vi "BMU诊断标定.vi"(5 "timeout":u32, 6 "Socket":dbl, 7 "通用配置?":bool, 8 "CAN端口":u16(ring), 9 "设备索引号":u16(ring), 10 "CAN卡类型":u32(ring)=21, 11 "从板号":u8=1) -> (3 "成功?":bool)   [LabVIEW 2013] (continued)
                n1293 = property on="配置文件版本" class="Str"("Disabled"=w1973) -> ()  [unwired: 2 in, 2 out]
                n1294 = property on="车架(牌)号" class="Str"("Disabled"=w1973) -> ()  [unwired: 2 in, 2 out]
                n1295 = property on="项目信息2" class="Clust (严格)"("DisabledEnum"=w1973) -> ()  [unwired: 2 in, 2 out]
                n1296 = property on="产品编号" class="Str"("Disabled"=w1973) -> ()  [unwired: 2 in, 2 out]
                n1297 = Not(x=w1977) -> (.not. x?=w1976:bool)
              }
              frame "产品编号" {
                w1990 = 2
                w1992 = FALSE
                n1298 = property on="项目信息" class="Tbl (严格)"("Disabled"=w1990) -> ()  [unwired: 2 in, 2 out]
                n1299 = property on="电池实际容量(A)" class="DigNum (严格)"("Disabled"=w1990) -> ()  [unwired: 2 in, 2 out]
                n1300 = property on="使用者" class="DigNum (严格)"("Disabled"=w1990) -> ()  [unwired: 2 in, 2 out]
                n1301 = Select(t=0, s=w1981, f=1) -> (s? t:f=w1980:i32)
                n1302 = property on="SOH(%)" class="DigNum (严格)"("Disabled"=w1990) -> ()  [unwired: 2 in, 2 out]
                n1303 = property on="电池额定容量(A)" class="DigNum (严格)"("Disabled"=w1990) -> ()  [unwired: 2 in, 2 out]
                n1304 = property on="SOC(%)" class="DigNum (严格)"("Disabled"=w1990) -> ()  [unwired: 2 in, 2 out]
                n1305 = property on="产品编号" class="Str"("Disabled"=w1980) -> ()  [unwired: 2 in, 2 out]
                n1306 = property on="项目信息2" class="Clust (严格)"("DisabledEnum"=w1980) -> ()  [unwired: 2 in, 2 out]
                n1307 = property on="系统时钟" class="Str"("Disabled"=w1990) -> ()  [unwired: 2 in, 2 out]
                n1308 = property on="配置文件版本" class="Str"("Disabled"=w1990) -> ()  [unwired: 2 in, 2 out]
                n1309 = property on="车架(牌)号" class="Str"("Disabled"=w1990) -> ()  [unwired: 2 in, 2 out]
                n1310 = property on="从板个数" class="DigNum (严格)"("NumText.BGColor"=u32 13816530) -> ()  [unwired: 2 in, 2 out]
                n1311 = global read "功能码全局.vi" "主板项目信息5"() -> (w1988:bool[])
                n1312 = global read "功能码全局.vi" "主板项目信息6"() -> (w1985:bool[])
                n1313 = Index Array(array=w1988, index=0 ("索引")) -> (element=w1987:bool)
                n1314 = Index Array(array=w1985, index=1 ("索引")) -> (element=w1984:bool)
                n1315 = Not(x=w1992) -> (.not. x?=w1991:bool)
              }
              frame "电压个数" {
                w2007 = 2
                w2009 = FALSE
                n1316 = local read "从板个数"() -> (w2006:dbl)
                n1317 = property on="从板个数" class="DigNum (严格)"("NumText.BGColor"=u32 6618880) -> ()  [unwired: 2 in, 2 out]
                n1318 = property on="电池实际容量(A)" class="DigNum (严格)"("Disabled"=w2007) -> ()  [unwired: 2 in, 2 out]
                n1319 = property on="使用者" class="DigNum (严格)"("Disabled"=w2007) -> ()  [unwired: 2 in, 2 out]
                n1320 = property on="SOH(%)" class="DigNum (严格)"("Disabled"=w2007) -> ()  [unwired: 2 in, 2 out]
                n1321 = property on="电池额定容量(A)" class="DigNum (严格)"("Disabled"=w2007) -> ()  [unwired: 2 in, 2 out]
                n1322 = property on="SOC(%)" class="DigNum (严格)"("Disabled"=w2007) -> ()  [unwired: 2 in, 2 out]
                n1323 = property on="系统时钟" class="Str"("Disabled"=w2007) -> ()  [unwired: 2 in, 2 out]
                n1324 = property on="配置文件版本" class="Str"("Disabled"=w2007) -> ()  [unwired: 2 in, 2 out]
                n1325 = property on="车架(牌)号" class="Str"("Disabled"=w2007) -> ()  [unwired: 2 in, 2 out]
                n1326 = property on="产品编号" class="Str"("Disabled"=w2007) -> ()  [unwired: 2 in, 2 out]
                n1327 = Select(t=0, s=w1996, f=1) -> (s? t:f=w1995:i32)
                n1328 = control-ref of="项目信息"() -> (w2005:refnum<vi>)
                n1329 = stacked-sequence {
                  tunnel: w2006 -> [_ w2016 w2026]
                  tunnel: w2005 -> [w2011 w2015 w2027]
                  frame #0 {
                    w2012 = 0
                    n1330 = Bundle(w2012, w2012) -> (w2014:cluster{i32, i32})  [unwired: 1 out]
                    n1331 = property class="Tbl (严格)"(reference=w2011, "Index Values"=w2014) -> (error out=w2013:errorcluster)  [unwired: 1 in, 1 out]
                    n1332 = call <vilib>:"Clear Errors.vi"("error in (no error)"=w2013) -> ()  [unwired: 7 out]
                  }
                  frame #1 {
                    n1333 = for {
                      N: 10 -> [_]
                      tunnel: w2015 -> [w2025]
                      tunnel: w2016 -> [w2020]
                      i -> [w2019]
                      n1334 = Compound Arithmetic op=ADD(0.0 ("值"), w2020, w2019) -> (w2022:dbl)
                      n1335 = Bundle(w2022, 0) -> (w2024:cluster{dbl, i32})  [unwired: 1 out]
                      n1336 = property class="Tbl (严格)"(reference=w2025, "Active Cell"=w2024, "Cell BG Color"=u32 16448250) -> ()  [unwired: 1 in, 2 out]
                    }
                  }
                  frame #2 {
                    n1337 = for {
                      N: w2026 -> [_]
                      tunnel: w2027 -> [w2028]
                      i -> [w2029]
                      n1338 = Bundle(w2029, 0) -> (w2033:cluster{i32, i32})  [unwired: 1 out]
                      n1339 = property class="Tbl (严格)"(reference=w2028, "Active Cell"=w2033, "Cell BG Color"=u32 6618880) -> (error out=w2030:errorcluster)  [unwired: 1 in, 1 out]
                      n1340 = call <vilib>:"Clear Errors.vi"("error in (no error)"=w2030) -> ()  [unwired: 7 out]
                    }
                  }
                }
                n1341 = property on="项目信息" class="Tbl (严格)"("Disabled"=w1995) -> ()  [unwired: 2 in, 2 out]
                n1342 = global read "功能码全局.vi" "主板项目信息5"() -> (w2003:bool[])
                n1343 = global read "功能码全局.vi" "主板项目信息6"() -> (w2001:bool[])
                n1344 = Index Array(array=w2003, index=1 ("索引")) -> (element=w2000:bool)
                n1345 = Index Array(array=w2001, index=2 ("索引")) -> (element=w1999:bool)
                n1346 = Not(x=w2009) -> (.not. x?=w2008:bool)
              }
              frame "通道电压数" {
                w2047 = 2
                w2049 = FALSE
                n1347 = property on="从板个数" class="DigNum (严格)"("NumText.BGColor"=u32 13816530) -> ()  [unwired: 2 in, 2 out]
                n1348 = property on="电池实际容量(A)" class="DigNum (严格)"("Disabled"=w2047) -> ()  [unwired: 2 in, 2 out]
                n1349 = property on="使用者" class="DigNum (严格)"("Disabled"=w2047) -> ()  [unwired: 2 in, 2 out]
                n1350 = property on="SOH(%)" class="DigNum (严格)"("Disabled"=w2047) -> ()  [unwired: 2 in, 2 out]
                n1351 = property on="电池额定容量(A)" class="DigNum (严格)"("Disabled"=w2047) -> ()  [unwired: 2 in, 2 out]
                n1352 = property on="SOC(%)" class="DigNum (严格)"("Disabled"=w2047) -> ()  [unwired: 2 in, 2 out]
                n1353 = local read "从板个数"() -> (w2045:dbl)
                n1354 = property on="系统时钟" class="Str"("Disabled"=w2047) -> ()  [unwired: 2 in, 2 out]
                n1355 = property on="配置文件版本" class="Str"("Disabled"=w2047) -> ()  [unwired: 2 in, 2 out]
                n1356 = property on="车架(牌)号" class="Str"("Disabled"=w2047) -> ()  [unwired: 2 in, 2 out]
                n1357 = property on="产品编号" class="Str"("Disabled"=w2047) -> ()  [unwired: 2 in, 2 out]
                n1358 = control-ref of="项目信息"() -> (w2046:refnum<vi>)
                n1359 = stacked-sequence {
                  tunnel: w2046 -> [w2056 w2059]
                  tunnel: w2045 -> [w2055 w2058]
                  frame #0 {
                    n1360 = Compound Arithmetic op=ADD(1.0 ("值"), w2055) -> (w2052:dbl)
                    n1361 = Bundle(w2052, 0) -> (w2054:cluster{dbl, i32})  [unwired: 1 out]
                    n1362 = property class="Tbl (严格)"(reference=w2056, "Index Values"=w2054) -> ()  [unwired: 1 in, 2 out]
                  }
                  frame #1 {
                    n1363 = for {
                      N: 20 -> [_]
                      tunnel: w2059 -> [w2067]
                      tunnel: w2058 -> [w2062]
                      i -> [w2061]
                      n1364 = Compound Arithmetic op=ADD(1.0 ("值"), w2062, w2061) -> (w2064:dbl)
                      n1365 = Bundle(w2064, 0) -> (w2066:cluster{dbl, i32})  [unwired: 1 out]
                      n1366 = property class="Tbl (严格)"(reference=w2067, "Active Cell"=w2066, "Cell BG Color"=u32 6618880) -> ()  [unwired: 1 in, 2 out]
                    }
                  }
                }
                n1367 = Select(t=0, s=w2035, f=1) -> (s? t:f=w2036:i32)
                n1368 = property on="项目信息" class="Tbl (严格)"("Disabled"=w2036) -> ()  [unwired: 2 in, 2 out]
                n1369 = global read "功能码全局.vi" "主板项目信息5"() -> (w2043:bool[])
                n1370 = global read "功能码全局.vi" "主板项目信息6"() -> (w2041:bool[])
                n1371 = Index Array(array=w2043, index=2 ("索引")) -> (element=w2040:bool)
                n1372 = Index Array(array=w2041, index=3 ("索引")) -> (element=w2039:bool)
                n1373 = Not(x=w2049) -> (.not. x?=w2048:bool)
              }
              frame "电压起始值" {
                w2081 = 2
                w2083 = FALSE
                n1374 = property on="从板个数" class="DigNum (严格)"("NumText.BGColor"=u32 13816530) -> ()  [unwired: 2 in, 2 out]
                n1375 = property on="电池实际容量(A)" class="DigNum (严格)"("Disabled"=w2081) -> ()  [unwired: 2 in, 2 out]
                n1376 = property on="使用者" class="DigNum (严格)"("Disabled"=w2081) -> ()  [unwired: 2 in, 2 out]
                n1377 = property on="SOH(%)" class="DigNum (严格)"("Disabled"=w2081) -> ()  [unwired: 2 in, 2 out]
                n1378 = property on="电池额定容量(A)" class="DigNum (严格)"("Disabled"=w2081) -> ()  [unwired: 2 in, 2 out]
                n1379 = property on="SOC(%)" class="DigNum (严格)"("Disabled"=w2081) -> ()  [unwired: 2 in, 2 out]
                n1380 = local read "从板个数"() -> (w2079:dbl)
                n1381 = property on="系统时钟" class="Str"("Disabled"=w2081) -> ()  [unwired: 2 in, 2 out]
                n1382 = property on="配置文件版本" class="Str"("Disabled"=w2081) -> ()  [unwired: 2 in, 2 out]
                n1383 = property on="车架(牌)号" class="Str"("Disabled"=w2081) -> ()  [unwired: 2 in, 2 out]
                n1384 = property on="产品编号" class="Str"("Disabled"=w2081) -> ()  [unwired: 2 in, 2 out]
                n1385 = control-ref of="项目信息"() -> (w2080:refnum<vi>)
                n1386 = stacked-sequence {
                  tunnel: w2080 -> [w2090 w2093 w2106]
                  tunnel: w2079 -> [w2089 w2092 w2105]
                  frame #0 {
                    n1387 = Compound Arithmetic op=ADD(21.0 ("值"), w2089) -> (w2086:dbl)
                    n1388 = Bundle(w2086, 0) -> (w2088:cluster{dbl, i32})  [unwired: 1 out]
                    n1389 = property class="Tbl (严格)"(reference=w2090, "Index Values"=w2088) -> ()  [unwired: 1 in, 2 out]
                  }
                  frame #1 {
                    n1390 = for {
                      N: 10 -> [_]
                      tunnel: w2093 -> [w2103]
                      tunnel: w2092 -> [w2098]
                      i -> [w2097]
                      n1391 = Multiply(x=w2098, y=2.0) -> (x*y=w2095:dbl)
                      n1392 = Compound Arithmetic op=ADD(21.0 ("值"), w2095, w2097) -> (w2100:dbl)
                      n1393 = Bundle(w2100, 0) -> (w2102:cluster{dbl, i32})  [unwired: 1 out]
                      n1394 = property class="Tbl (严格)"(reference=w2103, "Active Cell"=w2102, "Cell BG Color"=u32 16448250) -> ()  [unwired: 1 in, 2 out]
                    }
                  }
                  frame #2 {
                    n1395 = Increment(x=w2105) -> (x+1=w2104:dbl)
                    n1396 = for {
                      N: w2104 -> [_]
                      tunnel: w2106 -> [w2114]
                      tunnel: w2105 -> [w2109]
                      i -> [w2108]
                      n1397 = Compound Arithmetic op=ADD(21.0 ("值"), w2109, w2108) -> (w2111:dbl)
                      n1398 = Bundle(w2111, 0) -> (w2113:cluster{dbl, i32})  [unwired: 1 out]
                      n1399 = property class="Tbl (严格)"(reference=w2114, "Active Cell"=w2113, "Cell BG Color"=u32 6618880) -> ()  [unwired: 1 in, 2 out]
                    }
                  }
                }
                n1400 = Select(t=0, s=w2070, f=1) -> (s? t:f=w2069:i32)
                n1401 = property on="项目信息" class="Tbl (严格)"("Disabled"=w2069) -> ()  [unwired: 2 in, 2 out]
                n1402 = global read "功能码全局.vi" "主板项目信息5"() -> (w2077:bool[])
                n1403 = global read "功能码全局.vi" "主板项目信息6"() -> (w2075:bool[])
                n1404 = Index Array(array=w2077, index=3 ("索引")) -> (element=w2073:bool)
                n1405 = Index Array(array=w2075, index=4 ("索引")) -> (element=w2074:bool)
                n1406 = Not(x=w2083) -> (.not. x?=w2082:bool)
              }
              frame "温度个数" {
                w2128 = 2
                w2130 = FALSE
                n1407 = property on="电池实际容量(A)" class="DigNum (严格)"("Disabled"=w2128) -> ()  [unwired: 2 in, 2 out]
                n1408 = property on="使用者" class="DigNum (严格)"("Disabled"=w2128) -> ()  [unwired: 2 in, 2 out]
                n1409 = property on="SOH(%)" class="DigNum (严格)"("Disabled"=w2128) -> ()  [unwired: 2 in, 2 out]
                n1410 = property on="电池额定容量(A)" class="DigNum (严格)"("Disabled"=w2128) -> ()  [unwired: 2 in, 2 out]
                n1411 = property on="SOC(%)" class="DigNum (严格)"("Disabled"=w2128) -> ()  [unwired: 2 in, 2 out]
                n1412 = local read "从板个数"() -> (w2126:dbl)
                n1413 = control-ref of="项目信息"() -> (w2127:refnum<vi>)
                n1414 = stacked-sequence {
                  tunnel: w2127 -> [w2135 w2138 w2145]
                  tunnel: w2126 -> [w2132 w2137 w2144]
                  frame #0 {
                    n1415 = Bundle("从板个数"=w2132, 0) -> (w2134:cluster{"从板个数":dbl, i32})  [unwired: 1 out]
                    n1416 = property class="Tbl (严格)"(reference=w2135, "Index Values"=w2134) -> ()  [unwired: 1 in, 2 out]
                  }
                  frame #1 {
                    n1417 = for {
                      N: 20 -> [_]
                      tunnel: w2138 -> [w2143]
                      tunnel: w2137 -> [_]
                      i -> [w2139]
                      n1418 = Bundle(w2139, 0) -> (w2142:cluster{i32, i32})  [unwired: 1 out]
                      n1419 = property class="Tbl (严格)"(reference=w2143, "Active Cell"=w2142, "Cell BG Color"=u32 16448250) -> ()  [unwired: 1 in, 2 out]
                    }
                  }
                  frame #2 {
                    n1420 = for {
                      N: w2144 -> [_]
                      tunnel: w2145 -> [w2152]
                      tunnel: w2144 -> [w2146]
                      i -> [w2147]
                      n1421 = Compound Arithmetic op=ADD(w2146, w2147) -> (w2149:dbl)
                      n1422 = Bundle(w2149, 0) -> (w2151:cluster{dbl, i32})  [unwired: 1 out]
                      n1423 = property class="Tbl (严格)"(reference=w2152, "Active Cell"=w2151, "Cell BG Color"=u32 6618880) -> ()  [unwired: 1 in, 2 out]
                    }
                  }
                }
                n1424 = property on="系统时钟" class="Str"("Disabled"=w2128) -> ()  [unwired: 2 in, 2 out]
                n1425 = property on="配置文件版本" class="Str"("Disabled"=w2128) -> ()  [unwired: 2 in, 2 out]
                n1426 = property on="车架(牌)号" class="Str"("Disabled"=w2128) -> ()  [unwired: 2 in, 2 out]
                n1427 = property on="产品编号" class="Str"("Disabled"=w2128) -> ()  [unwired: 2 in, 2 out]
                n1428 = property on="从板个数" class="DigNum (严格)"("NumText.BGColor"=u32 13816530) -> ()  [unwired: 2 in, 2 out]
                n1429 = Select(t=0, s=w2117, f=1) -> (s? t:f=w2116:i32)
                n1430 = property on="项目信息" class="Tbl (严格)"("Disabled"=w2116) -> ()  [unwired: 2 in, 2 out]
                n1431 = global read "功能码全局.vi" "主板项目信息5"() -> (w2124:bool[])
                n1432 = global read "功能码全局.vi" "主板项目信息6"() -> (w2122:bool[])
                n1433 = Index Array(array=w2124, index=4 ("索引")) -> (element=w2120:bool)
                n1434 = Index Array(array=w2122, index=5 ("索引")) -> (element=w2121:bool)
                n1435 = Not(x=w2130) -> (.not. x?=w2129:bool)
              }
              frame "温度起始值" {
                w2166 = 2
                w2168 = FALSE
                n1436 = property on="电池实际容量(A)" class="DigNum (严格)"("Disabled"=w2166) -> ()  [unwired: 2 in, 2 out]
                n1437 = property on="使用者" class="DigNum (严格)"("Disabled"=w2166) -> ()  [unwired: 2 in, 2 out]
                n1438 = property on="SOH(%)" class="DigNum (严格)"("Disabled"=w2166) -> ()  [unwired: 2 in, 2 out]
                n1439 = property on="电池额定容量(A)" class="DigNum (严格)"("Disabled"=w2166) -> ()  [unwired: 2 in, 2 out]
                n1440 = property on="SOC(%)" class="DigNum (严格)"("Disabled"=w2166) -> ()  [unwired: 2 in, 2 out]
                n1441 = local read "从板个数"() -> (w2164:dbl)
                n1442 = property on="系统时钟" class="Str"("Disabled"=w2166) -> ()  [unwired: 2 in, 2 out]
                n1443 = property on="配置文件版本" class="Str"("Disabled"=w2166) -> ()  [unwired: 2 in, 2 out]
                n1444 = property on="车架(牌)号" class="Str"("Disabled"=w2166) -> ()  [unwired: 2 in, 2 out]
                n1445 = property on="产品编号" class="Str"("Disabled"=w2166) -> ()  [unwired: 2 in, 2 out]
                n1446 = control-ref of="项目信息"() -> (w2165:refnum<vi>)
                n1447 = stacked-sequence {
                  tunnel: w2165 -> [w2177 w2180 w2193]
                  tunnel: w2164 -> [w2170 w2179 w2192]
                  frame #0 {
                    n1448 = Multiply(x=w2170, y=3.0) -> (x*y=w2172:dbl)
                    n1449 = Compound Arithmetic op=ADD(23.0 ("值"), w2172) -> (w2174:dbl)
                    n1450 = Bundle(w2174, 0) -> (w2176:cluster{dbl, i32})  [unwired: 1 out]
                    n1451 = property class="Tbl (严格)"(reference=w2177, "Index Values"=w2176) -> ()  [unwired: 1 in, 2 out]
                  }
                  frame #1 {
                    n1452 = for {
                      N: 10 -> [_]
                      tunnel: w2180 -> [w2190]
                      tunnel: w2179 -> [w2185]
                      i -> [w2184]
                      n1453 = Multiply(x=4.0, y=w2185) -> (x*y=w2182:dbl)
                      n1454 = Compound Arithmetic op=ADD(24.0 ("值"), w2182, w2184) -> (w2187:dbl)
                      n1455 = Bundle(w2187, 0) -> (w2189:cluster{dbl, i32})  [unwired: 1 out]
                      n1456 = property class="Tbl (严格)"(reference=w2190, "Active Cell"=w2189, "Cell BG Color"=u32 16448250) -> ()  [unwired: 1 in, 2 out]
                    }
                  }
                  frame #2 {
                    n1457 = Increment(x=w2192) -> (x+1=w2191:dbl)
                    n1458 = for {
                      N: w2191 -> [_]
                      tunnel: w2193 -> [w2203]
                      tunnel: w2192 -> [w2198]
                      i -> [w2197]
                      n1459 = Multiply(x=3.0, y=w2198) -> (x*y=w2195:dbl)
                      n1460 = Compound Arithmetic op=ADD(23.0 ("值"), w2195, w2197) -> (w2200:dbl)
                      n1461 = Bundle(w2200, 0) -> (w2202:cluster{dbl, i32})  [unwired: 1 out]
                      n1462 = property class="Tbl (严格)"(reference=w2203, "Active Cell"=w2202, "Cell BG Color"=u32 6618880) -> ()  [unwired: 1 in, 2 out]
                    }
                  }
                }
                n1463 = Select(t=0, s=w2155, f=1) -> (s? t:f=w2154:i32)
                n1464 = property on="从板个数" class="DigNum (严格)"("NumText.BGColor"=u32 13816530) -> ()  [unwired: 2 in, 2 out]
                n1465 = property on="项目信息" class="Tbl (严格)"("Disabled"=w2154) -> ()  [unwired: 2 in, 2 out]
                n1466 = global read "功能码全局.vi" "主板项目信息5"() -> (w2162:bool[])
                n1467 = global read "功能码全局.vi" "主板项目信息6"() -> (w2160:bool[])
                n1468 = Index Array(array=w2162, index=5 ("索引")) -> (element=w2159:bool)
                n1469 = Index Array(array=w2160, index=6 ("索引")) -> (element=w2158:bool)
                n1470 = Not(x=w2168) -> (.not. x?=w2167:bool)
              }
              frame "保险位置" {
                w2216 = 2
                w2218 = FALSE
                n1471 = property on="电池实际容量(A)" class="DigNum (严格)"("Disabled"=w2216) -> ()  [unwired: 2 in, 2 out]
                n1472 = property on="使用者" class="DigNum (严格)"("Disabled"=w2216) -> ()  [unwired: 2 in, 2 out]
                n1473 = property on="SOH(%)" class="DigNum (严格)"("Disabled"=w2216) -> ()  [unwired: 2 in, 2 out]
                n1474 = property on="电池额定容量(A)" class="DigNum (严格)"("Disabled"=w2216) -> ()  [unwired: 2 in, 2 out]
                n1475 = property on="SOC(%)" class="DigNum (严格)"("Disabled"=w2216) -> ()  [unwired: 2 in, 2 out]
                n1476 = local read "从板个数"() -> (w2214:dbl)
                n1477 = property on="系统时钟" class="Str"("Disabled"=w2216) -> ()  [unwired: 2 in, 2 out]
                n1478 = property on="配置文件版本" class="Str"("Disabled"=w2216) -> ()  [unwired: 2 in, 2 out]
                n1479 = property on="车架(牌)号" class="Str"("Disabled"=w2216) -> ()  [unwired: 2 in, 2 out]
                n1480 = property on="产品编号" class="Str"("Disabled"=w2216) -> ()  [unwired: 2 in, 2 out]
                n1481 = control-ref of="项目信息"() -> (w2215:refnum<vi>)
                n1482 = stacked-sequence {
                  tunnel: w2215 -> [w2227 w2230]
                  tunnel: w2214 -> [w2220 w2229]
                  frame #0 {
                    n1483 = Multiply(x=w2220, y=4.0) -> (x*y=w2222:dbl)
                    n1484 = Compound Arithmetic op=ADD(24.0 ("值"), w2222) -> (w2224:dbl)
                    n1485 = Bundle(w2224, 0) -> (w2226:cluster{dbl, i32})  [unwired: 1 out]
                    n1486 = property class="Tbl (严格)"(reference=w2227, "Index Values"=w2226) -> ()  [unwired: 1 in, 2 out]
                  }
                  frame #1 {
                    n1487 = for {
                      N: 20 -> [_]
                      tunnel: w2230 -> [w2240]
                      tunnel: w2229 -> [w2235]
                      i -> [w2234]
                      n1488 = Multiply(x=4.0, y=w2235) -> (x*y=w2232:dbl)
                      n1489 = Compound Arithmetic op=ADD(24.0 ("值"), w2232, w2234) -> (w2237:dbl)
                      n1490 = Bundle(w2237, 0) -> (w2239:cluster{dbl, i32})  [unwired: 1 out]
                      n1491 = property class="Tbl (严格)"(reference=w2240, "Active Cell"=w2239, "Cell BG Color"=u32 6618880) -> ()  [unwired: 1 in, 2 out]
                    }
                  }
                }
                n1492 = property on="从板个数" class="DigNum (严格)"("NumText.BGColor"=u32 13816530) -> ()  [unwired: 2 in, 2 out]
                n1493 = Select(t=0, s=w2207, f=1) -> (s? t:f=w2205:i32)
                n1494 = global read "功能码全局.vi" "主板项目信息4"() -> (w2212:bool[])
                n1495 = property on="项目信息" class="Tbl (严格)"("Disabled"=w2205) -> ()  [unwired: 2 in, 2 out]
                n1496 = Index Array(array=w2212, index #1=5 ("索引"), index #2=6 ("索引")) -> (element #1=w2210:bool, element #2=w2209:bool)
                n1497 = Not(x=w2218) -> (.not. x?=w2217:bool)
              }
              frame "SOC" {
                w2251 = 2
                w2253 = FALSE
                n1498 = property on="电池实际容量(A)" class="DigNum (严格)"("Disabled"=w2251) -> ()  [unwired: 2 in, 2 out]
                n1499 = property on="使用者" class="DigNum (严格)"("Disabled"=w2251) -> ()  [unwired: 2 in, 2 out]
                n1500 = property on="SOH(%)" class="DigNum (严格)"("Disabled"=w2251) -> ()  [unwired: 2 in, 2 out]
                n1501 = property on="电池额定容量(A)" class="DigNum (严格)"("Disabled"=w2251) -> ()  [unwired: 2 in, 2 out]
                n1502 = property on="从板个数" class="DigNum (严格)"("NumText.BGColor"=u32 13816530) -> ()  [unwired: 2 in, 2 out]
                n1503 = property on="系统时钟" class="Str"("Disabled"=w2251) -> ()  [unwired: 2 in, 2 out]
                n1504 = property on="配置文件版本" class="Str"("Disabled"=w2251) -> ()  [unwired: 2 in, 2 out]
                n1505 = property on="车架(牌)号" class="Str"("Disabled"=w2251) -> ()  [unwired: 2 in, 2 out]
                n1506 = property on="项目信息" class="Tbl (严格)"("Disabled"=w2251) -> ()  [unwired: 2 in, 2 out]
                n1507 = property on="产品编号" class="Str"("Disabled"=w2251) -> ()  [unwired: 2 in, 2 out]
                n1508 = Select(t=0, s=w2243, f=0) -> (s? t:f=w2242:i32)
                n1509 = property on="SOC(%)" class="DigNum (严格)"("Disabled"=w2242) -> ()  [unwired: 2 in, 2 out]
                n1510 = property on="项目信息2" class="Clust (严格)"("DisabledEnum"=w2242) -> ()  [unwired: 2 in, 2 out]
                n1511 = global read "功能码全局.vi" "主板项目信息7"() -> (w2249:bool[])
                n1512 = Index Array(array=w2249, index #1=2 ("索引"), index #2=5 ("索引")) -> (element #1=w2247:bool, element #2=w2246:bool)
                n1513 = Not(x=w2253) -> (.not. x?=w2252:bool)
              }
              frame "电池额定实际容量" {
                w2265 = 2
                w2267 = FALSE
                n1514 = property on="使用者" class="DigNum (严格)"("Disabled"=w2265) -> ()  [unwired: 2 in, 2 out]
                n1515 = property on="SOH(%)" class="DigNum (严格)"("Disabled"=w2265) -> ()  [unwired: 2 in, 2 out]
                n1516 = property on="SOC(%)" class="DigNum (严格)"("Disabled"=w2265) -> ()  [unwired: 2 in, 2 out]
                n1517 = property on="从板个数" class="DigNum (严格)"("NumText.BGColor"=u32 13816530) -> ()  [unwired: 2 in, 2 out]
                n1518 = property on="系统时钟" class="Str"("Disabled"=w2265) -> ()  [unwired: 2 in, 2 out]
                n1519 = property on="配置文件版本" class="Str"("Disabled"=w2265) -> ()  [unwired: 2 in, 2 out]
                n1520 = property on="车架(牌)号" class="Str"("Disabled"=w2265) -> ()  [unwired: 2 in, 2 out]
                n1521 = property on="项目信息" class="Tbl (严格)"("Disabled"=w2265) -> ()  [unwired: 2 in, 2 out]
                n1522 = property on="产品编号" class="Str"("Disabled"=w2265) -> ()  [unwired: 2 in, 2 out]
                n1523 = Select(t=0, s=w2257, f=1) -> (s? t:f=w2256:i32)
                n1524 = property on="电池实际容量(A)" class="DigNum (严格)"("Disabled"=w2256) -> ()  [unwired: 2 in, 2 out]
                n1525 = property on="电池额定容量(A)" class="DigNum (严格)"("Disabled"=w2256) -> ()  [unwired: 2 in, 2 out]
                n1526 = property on="项目信息2" class="Clust (严格)"("DisabledEnum"=w2256) -> ()  [unwired: 2 in, 2 out]
                n1527 = global read "功能码全局.vi" "主板项目信息7"() -> (w2263:bool[])
                n1528 = Index Array(array=w2263, index #1=3 ("索引"), index #2=6 ("索引")) -> (element #1=w2261:bool, element #2=w2260:bool)
                n1529 = Not(x=w2267) -> (.not. x?=w2266:bool)
              }
              frame "配置文件版本" {
                w2280 = 2
                w2282 = FALSE
                n1530 = property on="使用者" class="DigNum (严格)"("Disabled"=w2280) -> ()  [unwired: 2 in, 2 out]
                n1531 = property on="SOH(%)" class="DigNum (严格)"("Disabled"=w2280) -> ()  [unwired: 2 in, 2 out]
                n1532 = property on="SOC(%)" class="DigNum (严格)"("Disabled"=w2280) -> ()  [unwired: 2 in, 2 out]
                n1533 = property on="电池实际容量(A)" class="DigNum (严格)"("Disabled"=w2280) -> ()  [unwired: 2 in, 2 out]
                n1534 = property on="从板个数" class="DigNum (严格)"("NumText.BGColor"=u32 13816530) -> ()  [unwired: 2 in, 2 out]
                n1535 = property on="电池额定容量(A)" class="DigNum (严格)"("Disabled"=w2280) -> ()  [unwired: 2 in, 2 out]
                n1536 = property on="系统时钟" class="Str"("Disabled"=w2280) -> ()  [unwired: 2 in, 2 out]
                n1537 = property on="车架(牌)号" class="Str"("Disabled"=w2280) -> ()  [unwired: 2 in, 2 out]
                n1538 = property on="项目信息" class="Tbl (严格)"("Disabled"=w2280) -> ()  [unwired: 2 in, 2 out]
                n1539 = property on="产品编号" class="Str"("Disabled"=w2280) -> ()  [unwired: 2 in, 2 out]
                n1540 = Select(t=0, s=w2271, f=1) -> (s? t:f=w2270:i32)
                n1541 = property on="项目信息2" class="Clust (严格)"("DisabledEnum"=w2270) -> ()  [unwired: 2 in, 2 out]
                n1542 = property on="配置文件版本" class="Str"("Disabled"=w2270) -> ()  [unwired: 2 in, 2 out]
                n1543 = global read "功能码全局.vi" "主板项目信息5"() -> (w2278:bool[])
                n1544 = global read "功能码全局.vi" "主板项目信息6"() -> (w2277:bool[])
                n1545 = Index Array(array=w2278, index=6 ("索引")) -> (element=w2275:bool)
                n1546 = Index Array(array=w2277, index=7 ("索引")) -> (element=w2274:bool)
                n1547 = Not(x=w2282) -> (.not. x?=w2281:bool)
              }
              frame "参数修改记录" {
                w2295 = 2
                w2297 = FALSE
                n1548 = property on="SOH(%)" class="DigNum (严格)"("Disabled"=w2295) -> ()  [unwired: 2 in, 2 out]
                n1549 = property on="SOC(%)" class="DigNum (严格)"("Disabled"=w2295) -> ()  [unwired: 2 in, 2 out]
                n1550 = property on="电池实际容量(A)" class="DigNum (严格)"("Disabled"=w2295) -> ()  [unwired: 2 in, 2 out]
                n1551 = property on="电池额定容量(A)" class="DigNum (严格)"("Disabled"=w2295) -> ()  [unwired: 2 in, 2 out]
                n1552 = property on="从板个数" class="DigNum (严格)"("NumText.BGColor"=u32 13816530) -> ()  [unwired: 2 in, 2 out]
                n1553 = property on="系统时钟" class="Str"("Disabled"=w2295) -> ()  [unwired: 2 in, 2 out]
                n1554 = property on="车架(牌)号" class="Str"("Disabled"=w2295) -> ()  [unwired: 2 in, 2 out]
                n1555 = property on="配置文件版本" class="Str"("Disabled"=w2295) -> ()  [unwired: 2 in, 2 out]
                n1556 = property on="项目信息" class="Tbl (严格)"("Disabled"=w2295) -> ()  [unwired: 2 in, 2 out]
                n1557 = property on="产品编号" class="Str"("Disabled"=w2295) -> ()  [unwired: 2 in, 2 out]
                n1558 = Select(t=0, s=w2286, f=1) -> (s? t:f=w2285:i32)
                n1559 = property on="使用者" class="DigNum (严格)"("Disabled"=w2285) -> ()  [unwired: 2 in, 2 out]
                n1560 = property on="项目信息2" class="Clust (严格)"("DisabledEnum"=w2285) -> ()  [unwired: 2 in, 2 out]
                n1561 = global read "功能码全局.vi" "主板项目信息7"() -> (w2292:bool[])
                n1562 = global read "功能码全局.vi" "主板项目信息5"() -> (w2293:bool[])
                n1563 = Index Array(array=w2292, index=0 ("索引")) -> (element=w2290:bool)
                n1564 = Index Array(array=w2293, index=7 ("索引")) -> (element=w2289:bool)
                n1565 = Not(x=w2297) -> (.not. x?=w2296:bool)
              }
              frame "车牌号" {
                w2310 = 2
                w2312 = FALSE
                n1566 = property on="SOH(%)" class="DigNum (严格)"("Disabled"=w2310) -> ()  [unwired: 2 in, 2 out]
                n1567 = property on="使用者" class="DigNum (严格)"("Disabled"=w2310) -> ()  [unwired: 2 in, 2 out]
                n1568 = property on="SOC(%)" class="DigNum (严格)"("Disabled"=w2310) -> ()  [unwired: 2 in, 2 out]
                n1569 = property on="电池实际容量(A)" class="DigNum (严格)"("Disabled"=w2310) -> ()  [unwired: 2 in, 2 out]
                n1570 = property on="电池额定容量(A)" class="DigNum (严格)"("Disabled"=w2310) -> ()  [unwired: 2 in, 2 out]
                n1571 = property on="从板个数" class="DigNum (严格)"("NumText.BGColor"=u32 13816530) -> ()  [unwired: 2 in, 2 out]
                n1572 = property on="系统时钟" class="Str"("Disabled"=w2310) -> ()  [unwired: 2 in, 2 out]
                n1573 = property on="配置文件版本" class="Str"("Disabled"=w2310) -> ()  [unwired: 2 in, 2 out]
                n1574 = property on="项目信息" class="Tbl (严格)"("Disabled"=w2310) -> ()  [unwired: 2 in, 2 out]
                n1575 = property on="产品编号" class="Str"("Disabled"=w2310) -> ()  [unwired: 2 in, 2 out]
                n1576 = Select(t=0, s=w2301, f=1) -> (s? t:f=w2300:i32)
                n1577 = property on="车架(牌)号" class="Str"("Disabled"=w2300) -> ()  [unwired: 2 in, 2 out]
                n1578 = property on="项目信息2" class="Clust (严格)"("DisabledEnum"=w2300) -> ()  [unwired: 2 in, 2 out]
                n1579 = global read "功能码全局.vi" "主板项目信息7"() -> (w2307:bool[])
                n1580 = global read "功能码全局.vi" "主板项目信息6"() -> (w2308:bool[])
                n1581 = Index Array(array=w2307, index=1 ("索引")) -> (element=w2305:bool)
                n1582 = Index Array(array=w2308, index=0 ("索引")) -> (element=w2304:bool)
                n1583 = Not(x=w2312) -> (.not. x?=w2311:bool)
              }
              frame "SOH" {
                w2324 = 2
                w2326 = FALSE
                n1584 = property on="使用者" class="DigNum (严格)"("Disabled"=w2324) -> ()  [unwired: 2 in, 2 out]
                n1585 = property on="SOC(%)" class="DigNum (严格)"("Disabled"=w2324) -> ()  [unwired: 2 in, 2 out]
                n1586 = property on="电池实际容量(A)" class="DigNum (严格)"("Disabled"=w2324) -> ()  [unwired: 2 in, 2 out]
                n1587 = property on="电池额定容量(A)" class="DigNum (严格)"("Disabled"=w2324) -> ()  [unwired: 2 in, 2 out]
                n1588 = property on="从板个数" class="DigNum (严格)"("NumText.BGColor"=u32 13816530) -> ()  [unwired: 2 in, 2 out]
                n1589 = property on="系统时钟" class="Str"("Disabled"=w2324) -> ()  [unwired: 2 in, 2 out]
                n1590 = property on="配置文件版本" class="Str"("Disabled"=w2324) -> ()  [unwired: 2 in, 2 out]
                n1591 = property on="项目信息" class="Tbl (严格)"("Disabled"=w2324) -> ()  [unwired: 2 in, 2 out]
                n1592 = property on="产品编号" class="Str"("Disabled"=w2324) -> ()  [unwired: 2 in, 2 out]
                n1593 = property on="车架(牌)号" class="Str"("Disabled"=w2324) -> ()  [unwired: 2 in, 2 out]
                n1594 = Select(t=0, s=w2316, f=1) -> (s? t:f=w2315:i32)
                n1595 = property on="项目信息2" class="Clust (严格)"("DisabledEnum"=w2315) -> ()  [unwired: 2 in, 2 out]
                n1596 = property on="SOH(%)" class="DigNum (严格)"("Disabled"=w2315) -> ()  [unwired: 2 in, 2 out]
                n1597 = global read "功能码全局.vi" "主板项目信息7"() -> (w2323:bool[])
                n1598 = Index Array(array=w2323, index #1=4 ("索引"), index #2=7 ("索引")) -> (element #1=w2320:bool, element #2=w2319:bool)
                n1599 = Not(x=w2326) -> (.not. x?=w2325:bool)
              }
              frame "SOC过低(2)", "SOC过高(2)", "SOH过低(2)", "充电电流过高(2)", "单体电压过低(2)", "单体电压过高(2)", "单组电压不均衡(2)", "单组温度不均衡(2)", "二级故障阀值", "放电电流过高(2)", "极柱温度过高(2)", "内阻过大(2)", "温度过低(2)", "温度过高(2)", "整组电压不均衡(2)", "整组温度不均衡(2)", "总电压过低(2)", "总电压过高(2)" {
                w2338 = FALSE
                n1600 = property on="从板个数" class="DigNum (严格)"("NumText.BGColor"=u32 13816530) -> ()  [unwired: 2 in, 2 out]
                n1601 = Select(t=0, s=w2330, f=1) -> (s? t:f=w2329:i32)
                n1602 = property on="一级故障 2" class="Clust (严格)"("DisabledEnum"=w2329) -> ()  [unwired: 2 in, 2 out]
                n1603 = global read "功能码全局.vi" "主板故障阀值9"() -> (w2336:bool[])
                n1604 = Index Array(array=w2336, index #1=3 ("索引"), index #2=6 ("索引")) -> (element #1=w2334:bool, element #2=w2333:bool)
                n1605 = Not(x=w2338) -> (.not. x?=w2339:bool)
              }
              frame "SOC过低(3)", "SOC过高(3)", "SOH过低(3)", "充电电流过高(3)", "单体电压过低(3)", "单体电压过高(3)", "单组电压不均衡(3)", "单组温度不均衡(3)", "放电电流过高(3)", "极柱温度过高(3)", "内阻过大(3)", "三级故障阀值", "温度过低(3)", "温度过高(3)", "整组电压不均衡(3)", "整组温度不均衡(3)", "总电压过低(3)", "总电压过高(3)" {
                w2352 = FALSE
                n1606 = property on="从板个数" class="DigNum (严格)"("NumText.BGColor"=u32 13816530) -> ()  [unwired: 2 in, 2 out]
                n1607 = Select(t=0, s=w2343, f=1) -> (s? t:f=w2342:i32)
                n1608 = property on="一级故障 3" class="Clust (严格)"("DisabledEnum"=w2342) -> ()  [unwired: 2 in, 2 out]
                n1609 = global read "功能码全局.vi" "主板故障阀值9"() -> (w2349:bool[])
                n1610 = Index Array(array=w2349, index #1=4 ("索引"), index #2=7 ("索引")) -> (element #1=w2347:bool, element #2=w2346:bool)
                n1611 = Not(x=w2352) -> (.not. x?=w2351:bool)
              }
              frame "SOC过低", "SOC过高", "SOH过低", "充电电流过高", "单体电压过低", "单体电压过高", "单组电压不均衡", "单组温度不均衡", "放电电流过高", "极柱温度过高", "内阻过大", "温度过低", "温度过高", "一级故障阀值", "整组电压不均衡", "整组温度不均衡", "总电压过低", "总电压过高" {
                w2365 = FALSE
                n1612 = Select(t=0, s=w2356, f=1) -> (s? t:f=w2355:i32)
                n1613 = property on="从板个数" class="DigNum (严格)"("NumText.BGColor"=u32 13816530) -> ()  [unwired: 2 in, 2 out]
                n1614 = property on="一级故障" class="Clust (严格)"("DisabledEnum"=w2355) -> ()  [unwired: 2 in, 2 out]
                n1615 = global read "功能码全局.vi" "主板故障阀值9"() -> (w2362:bool[])
                n1616 = Index Array(array=w2362, index #1=2 ("索引"), index #2=5 ("索引")) -> (element #1=w2360:bool, element #2=w2359:bool)
                n1617 = Not(x=w2365) -> (.not. x?=w2364:bool)
              }
              frame "充电控制参数", "电流步长", "最大允许充电电流", "最大允许充电温度", "最大允许单体电压", "最大允许总电压", "最小允许充电电流", "最小允许充电温度", "最小允许单体电压" {
                w2368 = 2
                w2379 = FALSE
                n1618 = property on="从板个数" class="DigNum (严格)"("NumText.BGColor"=u32 13816530) -> ()  [unwired: 2 in, 2 out]
                n1619 = property on="风机开启温度" class="DigNum (严格)"("Disabled"=w2368) -> ()  [unwired: 2 in, 2 out]
                n1620 = property on="风机关闭温度" class="DigNum (严格)"("Disabled"=w2368) -> ()  [unwired: 2 in, 2 out]
                n1621 = property on="加热开启温度" class="DigNum (严格)"("Disabled"=w2368) -> ()  [unwired: 2 in, 2 out]
                n1622 = property on="加热关闭温度" class="DigNum (严格)"("Disabled"=w2368) -> ()  [unwired: 2 in, 2 out]
                n1623 = property on="风机开启温差" class="DigNum (严格)"("Disabled"=w2368) -> ()  [unwired: 2 in, 2 out]
                n1624 = property on="风机关闭温差" class="DigNum (严格)"("Disabled"=w2368) -> ()  [unwired: 2 in, 2 out]
                n1625 = property on="加热控制参数" class="Clust (严格)"("DisabledEnum"=w2368) -> ()  [unwired: 2 in, 2 out]
                n1626 = Select(t=0, s=w2370, f=1) -> (s? t:f=w2369:i32)
                n1627 = property on="最大允许总电压" class="DigNum (严格)"("Disabled"=w2369) -> ()  [unwired: 2 in, 2 out]
                n1628 = property on="最大允许充电温度" class="DigNum (严格)"("Disabled"=w2369) -> ()  [unwired: 2 in, 2 out]
                n1629 = property on="最小允许充电温度" class="DigNum (严格)"("Disabled"=w2369) -> ()  [unwired: 2 in, 2 out]
                n1630 = property on="电流步长" class="DigNum (严格)"("Disabled"=w2369) -> ()  [unwired: 2 in, 2 out]
                n1631 = property on="最大允许单体电压" class="DigNum (严格)"("Disabled"=w2369) -> ()  [unwired: 2 in, 2 out]
                n1632 = property on="最小允许单体电压" class="DigNum (严格)"("Disabled"=w2369) -> ()  [unwired: 2 in, 2 out]
                n1633 = property on="最大允许充电电流" class="DigNum (严格)"("Disabled"=w2369) -> ()  [unwired: 2 in, 2 out]
                n1634 = property on="最小允许充电电流" class="DigNum (严格)"("Disabled"=w2369) -> ()  [unwired: 2 in, 2 out]
                n1635 = global read "功能码全局.vi" "主板控制类信息10"() -> (w2376:bool[])
                n1636 = Index Array(array=w2376, index #1=5 ("索引"), index #2=7 ("索引")) -> (element #1=w2374:bool, element #2=w2373:bool)
                n1637 = Not(x=w2379) -> (.not. x?=w2378:bool)
              }
              frame "风机关闭温差", "风机关闭温度", "风机开启温差", "风机开启温度", "加热关闭温差", "加热关闭温度", "加热开启温度", "加热控制参数" {
                w2391 = 2
                w2393 = FALSE
                n1638 = Select(t=0, s=w2383, f=1) -> (s? t:f=w2382:i32)
                n1639 = property on="从板个数" class="DigNum (严格)"("NumText.BGColor"=u32 13816530) -> ()  [unwired: 2 in, 2 out]
                n1640 = property on="加热控制参数" class="Clust (严格)"("DisabledEnum"=w2382) -> ()  [unwired: 2 in, 2 out]
                n1641 = property on="风机开启温度" class="DigNum (严格)"("Disabled"=w2382) -> ()  [unwired: 2 in, 2 out]
                n1642 = property on="风机关闭温度" class="DigNum (严格)"("Disabled"=w2382) -> ()  [unwired: 2 in, 2 out]
                n1643 = property on="加热开启温度" class="DigNum (严格)"("Disabled"=w2382) -> ()  [unwired: 2 in, 2 out]
                n1644 = property on="加热关闭温度" class="DigNum (严格)"("Disabled"=w2382) -> ()  [unwired: 2 in, 2 out]
                n1645 = property on="风机开启温差" class="DigNum (严格)"("Disabled"=w2382) -> ()  [unwired: 2 in, 2 out]
                n1646 = property on="风机关闭温差" class="DigNum (严格)"("Disabled"=w2382) -> ()  [unwired: 2 in, 2 out]
                n1647 = property on="最大允许总电压" class="DigNum (严格)"("Disabled"=w2391) -> ()  [unwired: 2 in, 2 out]
                n1648 = property on="最大允许充电温度" class="DigNum (严格)"("Disabled"=w2391) -> ()  [unwired: 2 in, 2 out]
                n1649 = property on="最小允许充电温度" class="DigNum (严格)"("Disabled"=w2391) -> ()  [unwired: 2 in, 2 out]
                n1650 = property on="电流步长" class="DigNum (严格)"("Disabled"=w2391) -> ()  [unwired: 2 in, 2 out]
                n1651 = property on="最大允许单体电压" class="DigNum (严格)"("Disabled"=w2391) -> ()  [unwired: 2 in, 2 out]
                n1652 = property on="最小允许单体电压" class="DigNum (严格)"("Disabled"=w2391) -> ()  [unwired: 2 in, 2 out]
                n1653 = property on="最大允许充电电流" class="DigNum (严格)"("Disabled"=w2391) -> ()  [unwired: 2 in, 2 out]
                n1654 = property on="最小允许充电电流" class="DigNum (严格)"("Disabled"=w2391) -> ()  [unwired: 2 in, 2 out]
                n1655 = global read "功能码全局.vi" "主板控制类信息10"() -> (w2389:bool[])
                n1656 = Index Array(array=w2389, index #1=4 ("索引"), index #2=6 ("索引")) -> (element #1=w2387:bool, element #2=w2386:bool)
                n1657 = Not(x=w2393) -> (.not. x?=w2392:bool)
              }
              frame "电池信息" {
                w2406 = FALSE
                n1658 = Select(t=0, s=w2397, f=1) -> (s? t:f=w2396:i32)
                n1659 = property on="电池串联" class="DigNum (严格)"("Disabled"=w2396) -> ()  [unwired: 2 in, 2 out]
                n1660 = property on="电池并联" class="DigNum (严格)"("Disabled"=w2396) -> ()  [unwired: 2 in, 2 out]
                n1661 = property on="电池包额定容量" class="DigNum (严格)"("Disabled"=w2396) -> ()  [unwired: 2 in, 2 out]
                n1662 = property on="电池包额定能量(kWh)" class="DigNum (严格)"("Disabled"=w2396) -> ()  [unwired: 2 in, 2 out]
                n1663 = property on="电池包额定总电压" class="DigNum (严格)"("Disabled"=w2396) -> ()  [unwired: 2 in, 2 out]
                n1664 = property on="实际容量" class="DigNum (严格)"("Disabled"=w2396) -> ()  [unwired: 2 in, 2 out]
                n1665 = property on="电池包组号" class="Str"("Disabled"=w2396) -> ()  [unwired: 2 in, 2 out]
                n1666 = property on="电池生产日期" class="Str"("Disabled"=w2396) -> ()  [unwired: 2 in, 2 out]
                n1667 = property on="电池厂家" class="Str"("Disabled"=w2396) -> ()  [unwired: 2 in, 2 out]
                n1668 = property on="电池类型" class="Str"("Disabled"=w2396) -> ()  [unwired: 2 in, 2 out]
                n1669 = property on="累计充电总安时" class="DigNum (严格)"("Disabled"=w2396) -> ()  [unwired: 2 in, 2 out]
                n1670 = property on="累计放电总安时" class="DigNum (严格)"("Disabled"=w2396) -> ()  [unwired: 2 in, 2 out]
                n1671 = property on="电池放空次数" class="DigNum (严格)"("Disabled"=w2396) -> ()  [unwired: 2 in, 2 out]
                n1672 = property on="电池充满次数" class="DigNum (严格)"("Disabled"=w2396) -> ()  [unwired: 2 in, 2 out]
                n1673 = property on="电池充电次数" class="DigNum (严格)"("Disabled"=w2396) -> ()  [unwired: 2 in, 2 out]
                n1674 = property on="电池信息" class="Clust (严格)"("DisabledEnum"=w2396) -> ()  [unwired: 2 in, 2 out]
                n1675 = global read "功能码全局.vi" "主板版本号11"() -> (w2403:bool[])
                n1676 = property on="从板个数" class="DigNum (严格)"("NumText.BGColor"=u32 13816530) -> ()  [unwired: 2 in, 2 out]
                n1677 = Index Array(array=w2403, index #1=0 ("索引"), index #2=1 ("索引")) -> (element #1=w2401:bool, element #2=w2400:bool)
                n1678 = Not(x=w2406) -> (.not. x?=w2405:bool)
              }
              frame "电池信息1" {
                w2418 = 2
                w2420 = FALSE
                n1679 = Select(t=0, s=w2410, f=1) -> (s? t:f=w2409:i32)
                n1680 = property on="电池信息" class="Clust (严格)"("DisabledEnum"=w2409) -> ()  [unwired: 2 in, 2 out]
                n1681 = property on="电池生产日期" class="Str"("Disabled"=w2409) -> ()  [unwired: 2 in, 2 out]
                n1682 = property on="电池厂家" class="Str"("Disabled"=w2409) -> ()  [unwired: 2 in, 2 out]
                n1683 = property on="电池类型" class="Str"("Disabled"=w2409) -> ()  [unwired: 2 in, 2 out]
                n1684 = property on="电池串联" class="DigNum (严格)"("Disabled"=w2409) -> ()  [unwired: 2 in, 2 out]
                n1685 = property on="电池并联" class="DigNum (严格)"("Disabled"=w2409) -> ()  [unwired: 2 in, 2 out]
                n1686 = property on="电池包额定容量" class="DigNum (严格)"("Disabled"=w2409) -> ()  [unwired: 2 in, 2 out]
                n1687 = property on="电池包额定能量(kWh)" class="DigNum (严格)"("Disabled"=w2409) -> ()  [unwired: 2 in, 2 out]
                n1688 = property on="电池包额定总电压" class="DigNum (严格)"("Disabled"=w2409) -> ()  [unwired: 2 in, 2 out]
                n1689 = property on="实际容量" class="DigNum (严格)"("Disabled"=w2409) -> ()  [unwired: 2 in, 2 out]
                n1690 = property on="累计充电总安时" class="DigNum (严格)"("Disabled"=w2418) -> ()  [unwired: 2 in, 2 out]
                n1691 = property on="累计放电总安时" class="DigNum (严格)"("Disabled"=w2418) -> ()  [unwired: 2 in, 2 out]
                n1692 = property on="电池放空次数" class="DigNum (严格)"("Disabled"=w2418) -> ()  [unwired: 2 in, 2 out]
                n1693 = property on="电池充满次数" class="DigNum (严格)"("Disabled"=w2418) -> ()  [unwired: 2 in, 2 out]
                n1694 = property on="电池充电次数" class="DigNum (严格)"("Disabled"=w2418) -> ()  [unwired: 2 in, 2 out]
                n1695 = property on="从板个数" class="DigNum (严格)"("NumText.BGColor"=u32 13816530) -> ()  [unwired: 2 in, 2 out]
                n1696 = property on="电池包组号" class="Str"("Disabled"=w2418) -> ()  [unwired: 2 in, 2 out]
                n1697 = global read "功能码全局.vi" "主板版本号11"() -> (w2416:bool[])
                n1698 = Index Array(array=w2416, index #1=0 ("索引"), index #2=1 ("索引")) -> (element #1=w2414:bool, element #2=w2413:bool)
                n1699 = Not(x=w2420) -> (.not. x?=w2419:bool)
              }
              frame "电池包组号" {
                w2432 = 2
                w2434 = FALSE
                n1700 = property on="电池生产日期" class="Str"("Disabled"=w2432) -> ()  [unwired: 2 in, 2 out]
                n1701 = property on="电池厂家" class="Str"("Disabled"=w2432) -> ()  [unwired: 2 in, 2 out]
                n1702 = property on="电池类型" class="Str"("Disabled"=w2432) -> ()  [unwired: 2 in, 2 out]
                n1703 = property on="电池串联" class="DigNum (严格)"("Disabled"=w2432) -> ()  [unwired: 2 in, 2 out]
                n1704 = property on="电池并联" class="DigNum (严格)"("Disabled"=w2432) -> ()  [unwired: 2 in, 2 out]
                n1705 = property on="电池包额定容量" class="DigNum (严格)"("Disabled"=w2432) -> ()  [unwired: 2 in, 2 out]
                n1706 = property on="电池包额定能量(kWh)" class="DigNum (严格)"("Disabled"=w2432) -> ()  [unwired: 2 in, 2 out]
                n1707 = property on="电池包额定总电压" class="DigNum (严格)"("Disabled"=w2432) -> ()  [unwired: 2 in, 2 out]
                n1708 = property on="实际容量" class="DigNum (严格)"("Disabled"=w2432) -> ()  [unwired: 2 in, 2 out]
                n1709 = property on="从板个数" class="DigNum (严格)"("NumText.BGColor"=u32 13816530) -> ()  [unwired: 2 in, 2 out]
                n1710 = property on="累计充电总安时" class="DigNum (严格)"("Disabled"=w2432) -> ()  [unwired: 2 in, 2 out]
                n1711 = property on="累计放电总安时" class="DigNum (严格)"("Disabled"=w2432) -> ()  [unwired: 2 in, 2 out]
                n1712 = property on="电池放空次数" class="DigNum (严格)"("Disabled"=w2432) -> ()  [unwired: 2 in, 2 out]
                n1713 = property on="电池充满次数" class="DigNum (严格)"("Disabled"=w2432) -> ()  [unwired: 2 in, 2 out]
                n1714 = property on="电池充电次数" class="DigNum (严格)"("Disabled"=w2432) -> ()  [unwired: 2 in, 2 out]
                n1715 = Select(t=0, s=w2424, f=1) -> (s? t:f=w2423:i32)
                n1716 = property on="电池包组号" class="Str"("Disabled"=w2423) -> ()  [unwired: 2 in, 2 out]
                n1717 = property on="电池信息" class="Clust (严格)"("DisabledEnum"=w2423) -> ()  [unwired: 2 in, 2 out]
                n1718 = global read "功能码全局.vi" "主板版本号11"() -> (w2430:bool[])
                n1719 = Index Array(array=w2430, index #1=0 ("索引"), index #2=1 ("索引")) -> (element #1=w2428:bool, element #2=w2427:bool)
                n1720 = Not(x=w2434) -> (.not. x?=w2433:bool)
              }
              frame "充放电安时" {
                w2446 = 2
                w2448 = FALSE
                n1721 = property on="电池生产日期" class="Str"("Disabled"=w2446) -> ()  [unwired: 2 in, 2 out]
                n1722 = property on="电池厂家" class="Str"("Disabled"=w2446) -> ()  [unwired: 2 in, 2 out]
                n1723 = property on="电池类型" class="Str"("Disabled"=w2446) -> ()  [unwired: 2 in, 2 out]
                n1724 = property on="电池串联" class="DigNum (严格)"("Disabled"=w2446) -> ()  [unwired: 2 in, 2 out]
                n1725 = property on="电池并联" class="DigNum (严格)"("Disabled"=w2446) -> ()  [unwired: 2 in, 2 out]
                n1726 = property on="电池包额定容量" class="DigNum (严格)"("Disabled"=w2446) -> ()  [unwired: 2 in, 2 out]
                n1727 = property on="电池包额定能量(kWh)" class="DigNum (严格)"("Disabled"=w2446) -> ()  [unwired: 2 in, 2 out]
                n1728 = property on="电池包额定总电压" class="DigNum (严格)"("Disabled"=w2446) -> ()  [unwired: 2 in, 2 out]
                n1729 = property on="实际容量" class="DigNum (严格)"("Disabled"=w2446) -> ()  [unwired: 2 in, 2 out]
                n1730 = property on="从板个数" class="DigNum (严格)"("NumText.BGColor"=u32 13816530) -> ()  [unwired: 2 in, 2 out]
                n1731 = Select(t=0, s=w2438, f=1) -> (s? t:f=w2437:i32)
                n1732 = property on="电池放空次数" class="DigNum (严格)"("Disabled"=w2446) -> ()  [unwired: 2 in, 2 out]
                n1733 = property on="电池充满次数" class="DigNum (严格)"("Disabled"=w2446) -> ()  [unwired: 2 in, 2 out]
                n1734 = property on="电池充电次数" class="DigNum (严格)"("Disabled"=w2446) -> ()  [unwired: 2 in, 2 out]
                n1735 = property on="电池包组号" class="Str"("Disabled"=w2446) -> ()  [unwired: 2 in, 2 out]
                n1736 = property on="累计充电总安时" class="DigNum (严格)"("Disabled"=w2437) -> ()  [unwired: 2 in, 2 out]
                n1737 = property on="累计放电总安时" class="DigNum (严格)"("Disabled"=w2437) -> ()  [unwired: 2 in, 2 out]
                n1738 = property on="电池信息" class="Clust (严格)"("DisabledEnum"=w2437) -> ()  [unwired: 2 in, 2 out]
                n1739 = global read "功能码全局.vi" "主板版本号11"() -> (w2444:bool[])
                n1740 = Index Array(array=w2444, index #1=0 ("索引"), index #2=1 ("索引")) -> (element #1=w2442:bool, element #2=w2441:bool)
                n1741 = Not(x=w2448) -> (.not. x?=w2447:bool)
              }
              frame "电池充放电次数" {
                w2460 = 2
                w2462 = FALSE
                n1742 = property on="从板个数" class="DigNum (严格)"("NumText.BGColor"=u32 13816530) -> ()  [unwired: 2 in, 2 out]
                n1743 = property on="电池生产日期" class="Str"("Disabled"=w2460) -> ()  [unwired: 2 in, 2 out]
                n1744 = property on="电池厂家" class="Str"("Disabled"=w2460) -> ()  [unwired: 2 in, 2 out]
                n1745 = property on="电池类型" class="Str"("Disabled"=w2460) -> ()  [unwired: 2 in, 2 out]
                n1746 = property on="电池串联" class="DigNum (严格)"("Disabled"=w2460) -> ()  [unwired: 2 in, 2 out]
                n1747 = property on="电池并联" class="DigNum (严格)"("Disabled"=w2460) -> ()  [unwired: 2 in, 2 out]
                n1748 = property on="电池包额定容量" class="DigNum (严格)"("Disabled"=w2460) -> ()  [unwired: 2 in, 2 out]
                n1749 = property on="电池包额定能量(kWh)" class="DigNum (严格)"("Disabled"=w2460) -> ()  [unwired: 2 in, 2 out]
                n1750 = property on="电池包额定总电压" class="DigNum (严格)"("Disabled"=w2460) -> ()  [unwired: 2 in, 2 out]
                n1751 = property on="实际容量" class="DigNum (严格)"("Disabled"=w2460) -> ()  [unwired: 2 in, 2 out]
                n1752 = Select(t=0, s=w2452, f=1) -> (s? t:f=w2451:i32)
                n1753 = property on="电池放空次数" class="DigNum (严格)"("Disabled"=w2451) -> ()  [unwired: 2 in, 2 out]
                n1754 = property on="电池充满次数" class="DigNum (严格)"("Disabled"=w2451) -> ()  [unwired: 2 in, 2 out]
                n1755 = property on="电池充电次数" class="DigNum (严格)"("Disabled"=w2451) -> ()  [unwired: 2 in, 2 out]
                n1756 = property on="累计充电总安时" class="DigNum (严格)"("Disabled"=w2460) -> ()  [unwired: 2 in, 2 out]
                n1757 = property on="累计放电总安时" class="DigNum (严格)"("Disabled"=w2460) -> ()  [unwired: 2 in, 2 out]
                n1758 = property on="电池信息" class="Clust (严格)"("DisabledEnum"=w2451) -> ()  [unwired: 2 in, 2 out]
                n1759 = property on="电池包组号" class="Str"("Disabled"=w2460) -> ()  [unwired: 2 in, 2 out]
                n1760 = global read "功能码全局.vi" "主板版本号11"() -> (w2458:bool[])
                n1761 = Index Array(array=w2458, index #1=0 ("索引"), index #2=1 ("索引")) -> (element #1=w2456:bool, element #2=w2455:bool)
                n1762 = Not(x=w2462) -> (.not. x?=w2461:bool)
              }
              frame "假", Default {
                w2467 = FALSE
                n1763 = Not(x=w2467) -> (.not. x?=w2466:bool)
              }
            }
            n1764 = property on="单个读取" class="Bool (严格)"("Visible"=w1950) -> ()  [unwired: 2 in, 2 out]
            n1765 = property on="单个写入" class="Bool (严格)"("Visible"=w1949) -> ()  [unwired: 2 in, 2 out]
            n1766 = local write "1"(w1957) -> ()
            n1767 = local write "1 2"(w1956) -> ()
            n1768 = local write "1 3"(w1955) -> ()
            n1769 = local write "1 4"(w1954) -> ()
            n1770 = local write "1 5"(w1953) -> ()
            n1771 = local write "1 11"(w1952) -> ()
            n1772 = local write "主板2"(w1958) -> ()
          }
          event "从板选项": Mouse Down {
            n1773 = event-data() -> ("CtlRef"=w2482:refnum<vi>)  [unwired: 8 out]
            n1774 = property class="Tree (严格)"(reference=w2482) -> ("Value"=w2481:string)  [unwired: 1 in, 2 out]
            n1775 = global read "功能码全局.vi" "主板监控2"() -> (w2472:bool[])
            n1776 = Index Array(array=w2472, index=6 ("索引")) -> (element=w2470:bool)
            n1777 = case shown="\"温度个数\"" w2481 {
